vi "read message.vi"(9 "continuation timeout (10000)":i32=10000, 10 "base timeout (5000)":i32=5000, 11 "tcp connection":refnum<k5>) -> (0 "error":errorcluster, 2 "Numeric":u8=2, 3 "message":string)   [LabVIEW 2016, in "websocket core.lvlib"]
uses:
  websocket core.lvlib
  lvlibtls/socket connection/lvlibretls connection.lvclass
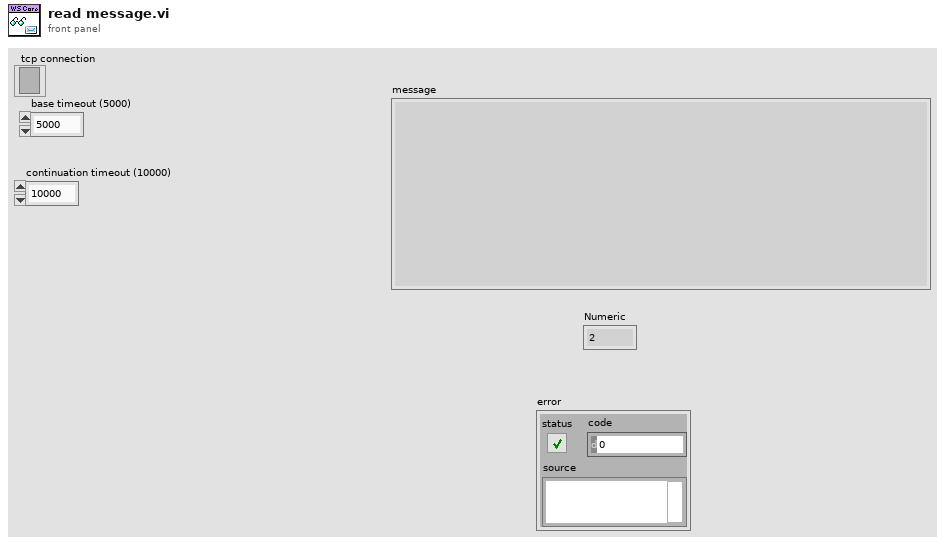
[diagram p1: front panel]
types:
  T1 = typedef "websocket core.lvlib/first byte header.ctl" = cluster{"fin":bool, "RSRV1":bool, "RSRV2":bool, "RSRV3":bool, "opcode":u8}
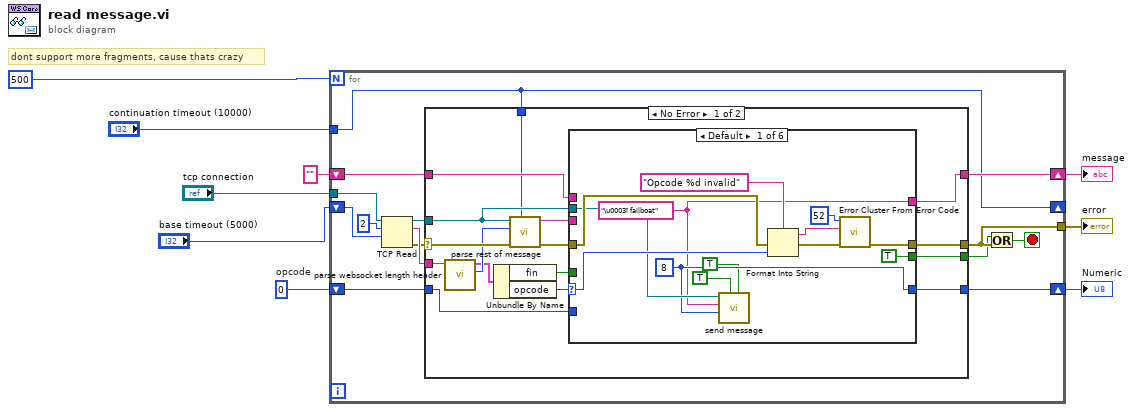
[diagram p0: block diagram]
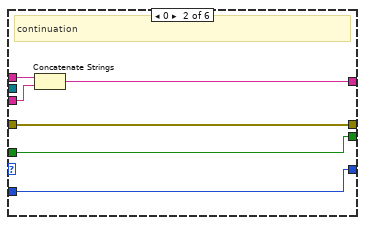
[diagram p2: hidden frame]
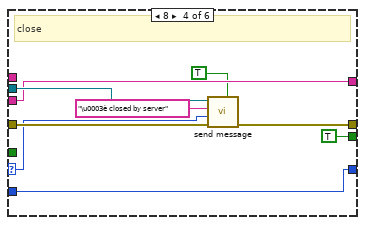
[diagram p4: hidden frame]
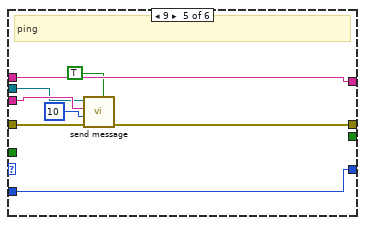
[diagram p5: hidden frame]
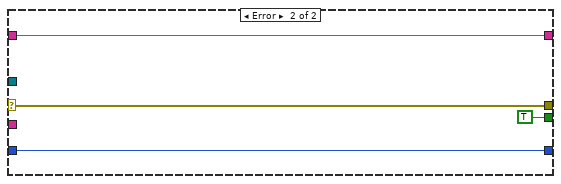
[diagram p7: hidden frame]
diagram:
  w8 = u8 0  # opcode
  # "dont support more fragments, cause thats crazy"
  n1 = for {
    N: 500 -> [_]
    tunnel: "tcp connection" -> [w20]
    tunnel: [w18] -> w6
    shift-right: [w16] -> w4
    shift-left: "" -> [w17]
    shift-right: [w14] -> w3
    shift-left: w8 -> [w15]
    shift-right: [w10] -> _
    shift-left: "base timeout (5000)" -> [w11]
    tunnel: "continuation timeout (10000)" -> [w10]
    stop <- w12 stop-if-true
    n2 = TCP Read(connection ID=w20, bytes to read=2, 9:w11) -> (connection ID out=w21:refnum<k5>, data out=w23:string, error out=w19:errorcluster)  [unwired: 2 in]
    n3 = case shown="No Error" w19 {
      selector: w19 -> [w39 w86]
      tunnel: w23 -> [w38 _]
      tunnel: w21 -> [w28 _]
      tunnel: [w35 w86] -> w18
      tunnel: w17 -> [w31 w85]
      tunnel: [w32 w85] -> w16
      tunnel: w15 -> [w25 w84]
      tunnel: [w26 w84] -> w14
      tunnel: [w27 TRUE] -> w13
      tunnel: w10 -> [w24 _]
      frame No Error {
        n4 = call "parse websocket length header.vi"("header string"=w38) -> ("mask(1)+length(7)"=w37:u8, "first byte"=w36:T1)  [unwired: 9 in]
        n5 = Unbundle By Name(w36) -> ("fin"=w29:bool, "opcode"=w33:u8)
        n6 = call "parse rest of message.vi"("continuation timeout ms (2000)"=w24, "error in"=w39, "mask(1)+length(7)"=w37, "lvlibretls connection in"=w28) -> ("error out"=w34:errorcluster, "unmasked data"=w30:string)  [unwired: 6 in]
        n7 = case shown="Default" w33 {
          selector: w33 -> [w47 _ w60 w67 _ _]
          tunnel: [w51 w56 w62 w69 w74 w80] -> w35
          tunnel: w34 -> [w52 w56 w62 w70 w78 w80]
          tunnel: [w41 w55 w61 w64 w79 w82] -> w32
          tunnel: w31 -> [_ w58 _ _ w79 w82]
          tunnel: w30 -> [_ w57 w61 w64 w76 _]
          tunnel: w29 -> [_ w53 w59 _ _ _]
          tunnel: w28 -> [w44 _ _ w71 w75 _]
          tunnel: [TRUE ("fin") w53 w59 TRUE _ _] -> w27
          tunnel: [w42 w54 w60 w66 w73 w81] -> w26
          tunnel: w25 -> [_ w54 _ w66 w73 w81]
          frame Default {
            w42 = u8 8 ("opcode")
            w41 = "\u0003ï failboat" ("data")
            n8 = call "send message.vi"("mask? (F)"=TRUE, "final fragment (T)"=TRUE, "opcode"=w42, "data"=w41, "lvlibretls connection in"=w44) -> ()  [unwired: 5 in, 2 out]
            n9 = Format Into String(format string="Opcode %d invalid", error in=w52, w47) -> (resulting string=w48:string, error out=w49:errorcluster)  [unwired: 1 in]
            n10 = call <vilib>:"Error Cluster From Error Code.vi"("error in (no error)"=w49, "error message (\"\")"=w48, "error code (0)"=52) -> ("error out"=w51:errorcluster)  [unwired: 6 in]
          }
          frame 0 {
            # "continuation"
            n11 = Concatenate Strings(w58, w57) -> (w55:string)
          }
          frame 1..7 {
            # "appdata"
          }
          frame 8 {
            # "close"
            n12 = call "send message.vi"("mask? (F)"=TRUE, "error in"=w70, "opcode"=w67, "data"="\u0003è closed by server", "lvlibretls connection in"=w71) -> ("error out"=w69:errorcluster)  [unwired: 5 in, 1 out]
          }
          frame 9 {
            # "ping"
            n13 = call "send message.vi"("mask? (F)"=TRUE, "error in"=w78, "opcode"=u8 10, "data"=w76, "lvlibretls connection in"=w75) -> ("error out"=w74:errorcluster)  [unwired: 5 in, 1 out]
          }
          frame 10 {
            # "pong, would only rx if app sends"
          }
        }
      }
      frame Error {
      }
    }
    n14 = Or(x=w13, y=w18) -> (x .or. y?=w12:bool)
  }
  "error" <- w6
  "message" <- w4
  "Numeric" <- w3
